vi "4.3_PH.vi"() -> ()   [LabVIEW 2023]
panel:
  out "n-ty":dbl
  in  "a1":dbl
  in  "q":dbl
  out "Suma n wyrazów":dbl
  in  "iloœæ kroków":dbl=1.0
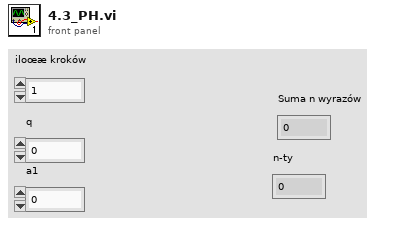
[diagram p1: front panel]
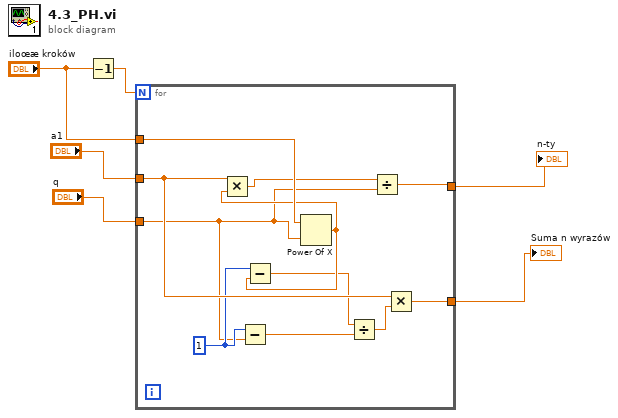
[diagram p0: block diagram]
diagram:
  n1 = Decrement(x="iloœæ kroków") -> (x-1=w3:dbl)
  n2 = for {
    N: w3 -> [_]
    tunnel: "q" -> [w8]
    tunnel: "a1" -> [w14]
    tunnel: "iloœæ kroków" -> [w17]
    tunnel: [w7] -> w5
    tunnel: [w10] -> w2
    w13 = 1
    n3 = Subtract(x=w13, y=w8) -> (x-y=w16:dbl)
    n4 = Power Of X(1:w8, 2:w17) -> (0:w12:dbl)
    n5 = Multiply(x=w14, y=w12) -> (x*y=w9:dbl)
    n6 = Subtract(x=w13, y=w12) -> (x-y=w11:dbl)
    n7 = Divide(x=w11, y=w16) -> (x/y=w15:dbl)
    n8 = Divide(x=w9, y=w8) -> (x/y=w7:dbl)
    n9 = Multiply(x=w14, y=w15) -> (x*y=w10:dbl)
  }
  "n-ty" <- w5
  "Suma n wyrazów" <- w2
